vi "FdxCmdTxCreateVLCvi.vi"(8 "error in":errorcluster, 9 "Input Cluster":T1 {"NetSelect" items=["FDX_TX_FRAME_DLY_A"=0, "FDX_TX_FRAME_DLY_B"=1, "FDX_TX_FRAME_BOTH "=3, "FDX_TX_FRAME_ONLY_A"=4, "FDX_TX_FRAME_ONLY_B "=5]}, 11 "InstrumentHandle_port in":u32) -> (0 "error out":errorcluster, 3 "InstrumentHandle_port out":u32)   [LabVIEW 2020, in "AIM664LV.lvlib"]
doc: "This function is used to setup a Virtual Link to transmit data. This is only a description of the Virtual Link specific parameters, which must be known by the system for transmitting. This function can be used only when the transmitter is not running."
uses:
  AIM664LV.lvlib
  AFDX_LibraryAdmin/FdxGlobalDllPath.vi
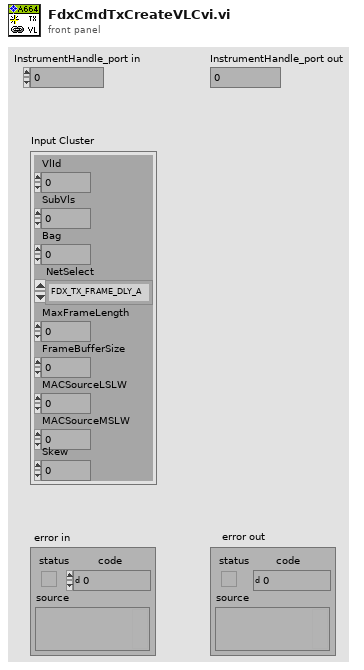
[diagram p1: front panel]
types:
  T1 = cluster{"VlId":u32, "SubVls":u32, "Bag":u32, "NetSelect":u32, "MaxFrameLength":u32, "FrameBufferSize":u32, "MACSourceLSLW":u32, "MACSourceMSLW":u32, "Skew":u32}
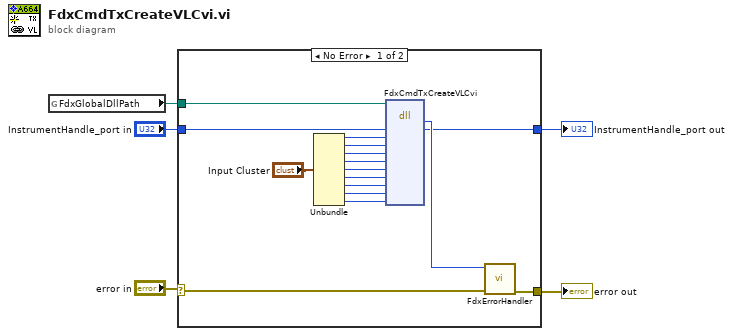
[diagram p0: block diagram]
diagram:
  n1 = global read "FdxGlobalDllPath.vi" "FdxGlobalDllPath"() -> (w3:path)
  n2 = case shown="No Error" "error in" {
    selector: "error in" -> [w20 w23]
    tunnel: [w21 w23] -> w5
    tunnel: w3 -> [w8 _]
    tunnel: "InstrumentHandle_port in" -> [w7 w22]
    tunnel: [w6 w22] -> w1
    frame No Error {
      n3 = Unbundle("Input Cluster") -> ("VlId"=w17:u32, "SubVls"=w16:u32, "Bag"=w15:u32, "NetSelect"=w14:u32, "MaxFrameLength"=w13:u32, "FrameBufferSize"=w12:u32, "MACSourceLSLW"=w11:u32, "MACSourceMSLW"=w10:u32, "Skew"=w9:u32)
      n4 = dll-call lib="aim_fdx.19.dll" fn="FdxCmdTxCreateVLCvi"(path in=w8, "InstrumentHandle"=w7, "VlId"=w17, "SubVls"=w16, "Bag"=w15, "NetSelect"=w14, "MaxFrameLength"=w13, "FrameBufferSize"=w12, "MACSourceLSLW"=w11, "MACSourceMSLW"=w10, "Skew"=w9) -> ("status"=w19:i32, "InstrumentHandle"=w6:u32)  [unwired: 11 in, 2 out]
      n5 = call "FdxErrorHandler.vi"("error in"=w20, "AIM Error"=w19) -> ("error out"=w21:errorcluster)  [unwired: 9 in]
    }
    frame Error {
    }
  }
  "error out" <- w5
  "InstrumentHandle_port out" <- w1
